vi "Arm Height Calculations.vi"(10 "Height Input":dbl) -> (1 "At Height?":bool)   [LabVIEW 2013]
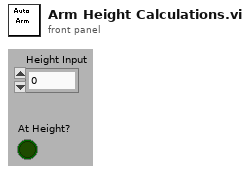
[diagram p1: front panel]
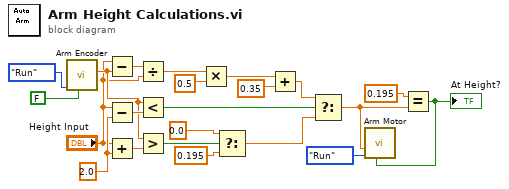
[diagram p0: block diagram]
diagram:
  w9 = 2.0 ("y")
  n1 = call "Arm Encoder.vi"("Reset Encoder?"=FALSE, "Mode"=enum16{"Init", "Run", "End"}."Run") -> ("Get Arm Encoder"=w6:dbl)  [unwired: 1 in, 8 out]
  n2 = Subtract(x="Height Input", y=w6) -> (x-y=w12:dbl)
  n3 = Subtract(x="Height Input", y=w9) -> (x-y=w10:dbl)
  n4 = Add(x="Height Input", y=w9) -> (x+y=w11:dbl)
  n5 = Divide(x=w12, y="Height Input") -> (x/y=w17:dbl)
  n6 = Less?(x=w6, y=w10) -> (x < y?=w19:bool)
  n7 = Greater?(x=w6, y=w11) -> (0:w22:bool)
  n8 = Multiply(x=w17, y=0.5) -> (x*y=w16:dbl)
  n9 = Select(t=0.0, s=w22, f=0.195 ("t")) -> (s? t:f=w18:dbl)
  n10 = Add(x=w16, y=0.35) -> (x+y=w14:dbl)
  n11 = Select(t=w14, s=w19, f=w18) -> (s? t:f=w2:dbl)
  n12 = Equal?(x=0.195, y=w2) -> (x = y?=w1:bool)
  "At Height?" <- w1
  n13 = call "Arm Motor.vi"("Stall Arm?"=w1, "Mode"=enum16{"Init", "Run", "End"}."Run", "Arm motor speed"=w2) -> ()  [unwired: 1 in, 8 out]
